vi "main5-2.vi"() -> ()   [LabVIEW 2018]
uses:
  <vilib>/Utility/file.llb/Write Delimited Spreadsheet (string).vi
panel:
  in  "备忘录保存路径":path
  out "光谱仪错误 2":errorcluster caption="光谱仪 R 错误"
  out "光谱仪错误":errorcluster caption="光谱仪 T 错误"
  in  "扫描模式":u16(ring)=2 items=["Norm/Hold", "Norm/Auto", "MID", "HIGH1", "HIGH2", "HIGH3", "Normal"]
  in  "终止波长":dbl=1542.0 caption="终止波长(nm)" format="%#_13g"
  in  "起始波长":dbl=1522.0 caption="起始波长(nm)" format="%#_13g"
  out "R中心波长-时间":waveform(dbl)(graph)
  out "T中心波长-时间":waveform(dbl)(graph)
  in  "T X dB":dbl=1.0 format="%#_13g"
  in  "保存路径R":path=path "C:/Users/Administrator/Desktop/超高温FBG实验程序/data/guangpuyi.txt" caption="R 光谱数据保存路径"
  in  "保存":bool
  in  "保存路径T":path=path "C:/Users/Administrator/Desktop/超高温FBG实验程序/data/guangpuyi.txt" caption="T 光谱数据保存路径"
  out "波峰带宽":dbl format="%.4f"
  out "Data X Value":dbl[](array[numeric]) format="%.4f"
  out "反射谱":T1(graph)
  out "R中心波长":dbl format="%.4f"
  out "波谷带宽":dbl format="%.4f"
  out "Data X Value":dbl[](array[numeric]) format="%.4f"
  out "采样点数":i32
  out "透射谱":T1(graph)
  out "T中心波长":dbl format="%.4f"
  in  "光谱仪 R":refnum<visa-resource-name>="光谱仪"
  in  "停止":bool
  in  "采集间隔":u32=30000 caption="采集间隔(ms)"
  in  "光谱仪 T":refnum<visa-resource-name>="光谱仪"
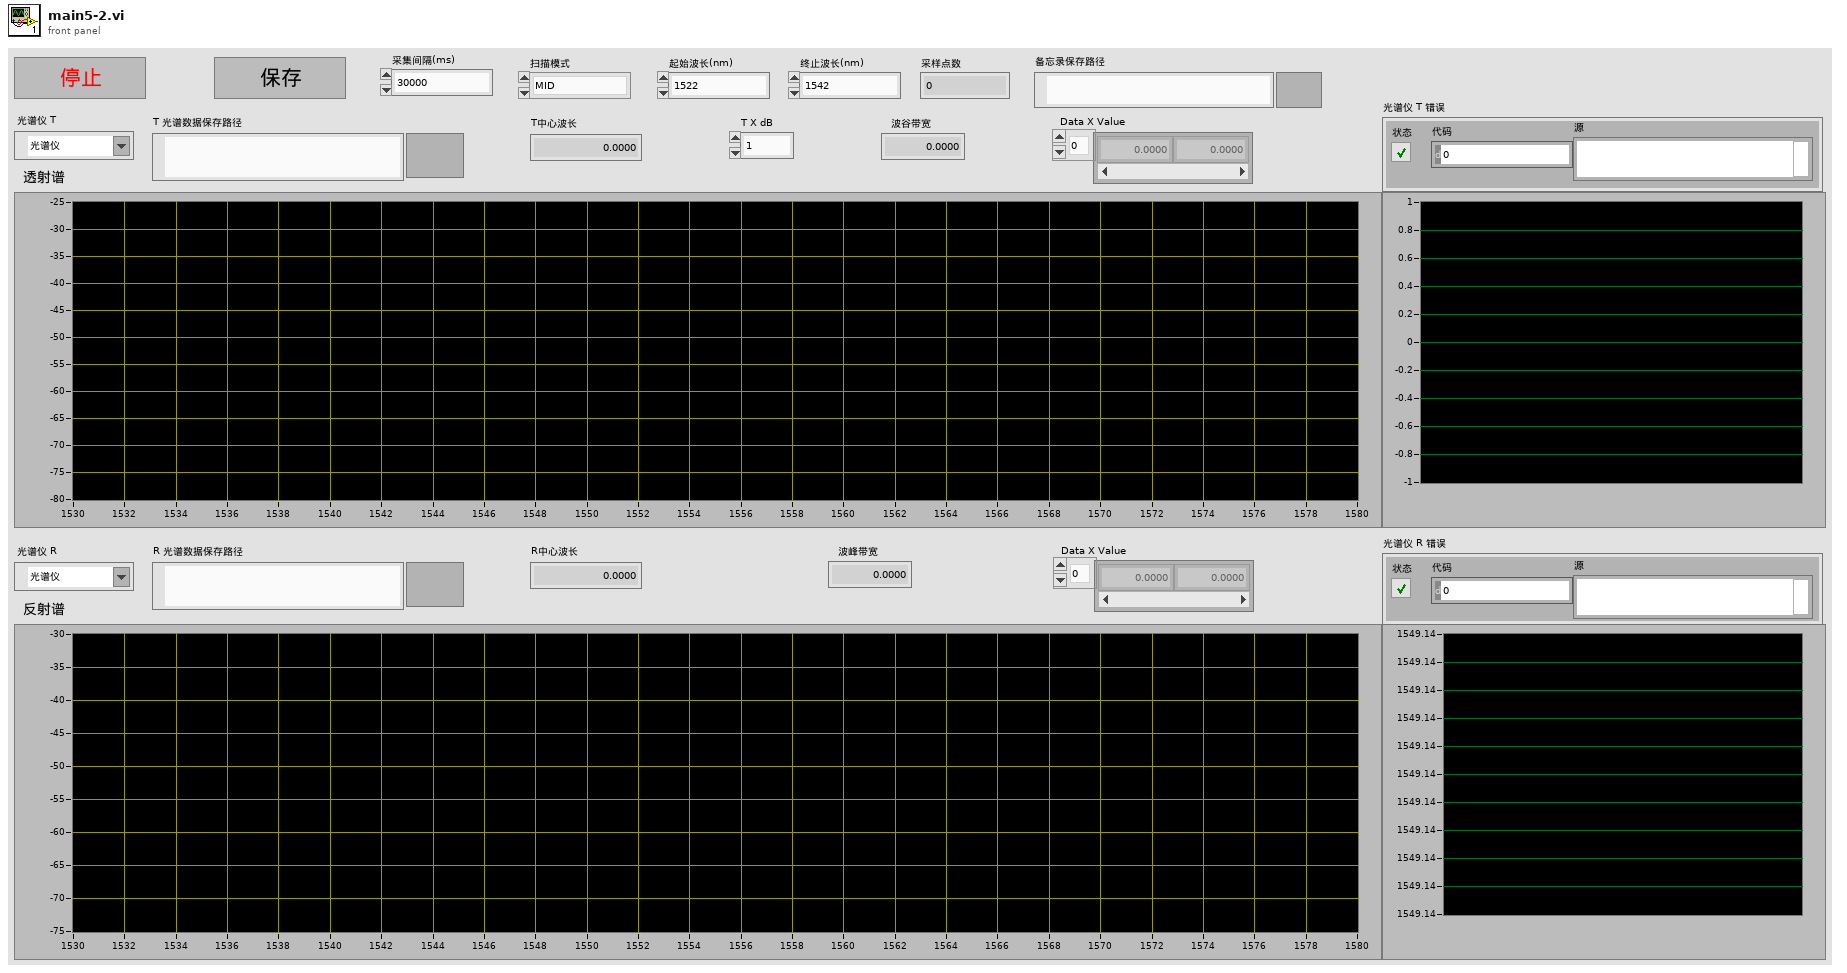
[diagram p1: front panel]
types:
  T1 = cluster{"Data X Value":dbl[], "Data Y Value":dbl[]}
  T2 = enum16{"open", "replace", "create", "open or create", "replace or create", "replace or create with confirmation"}
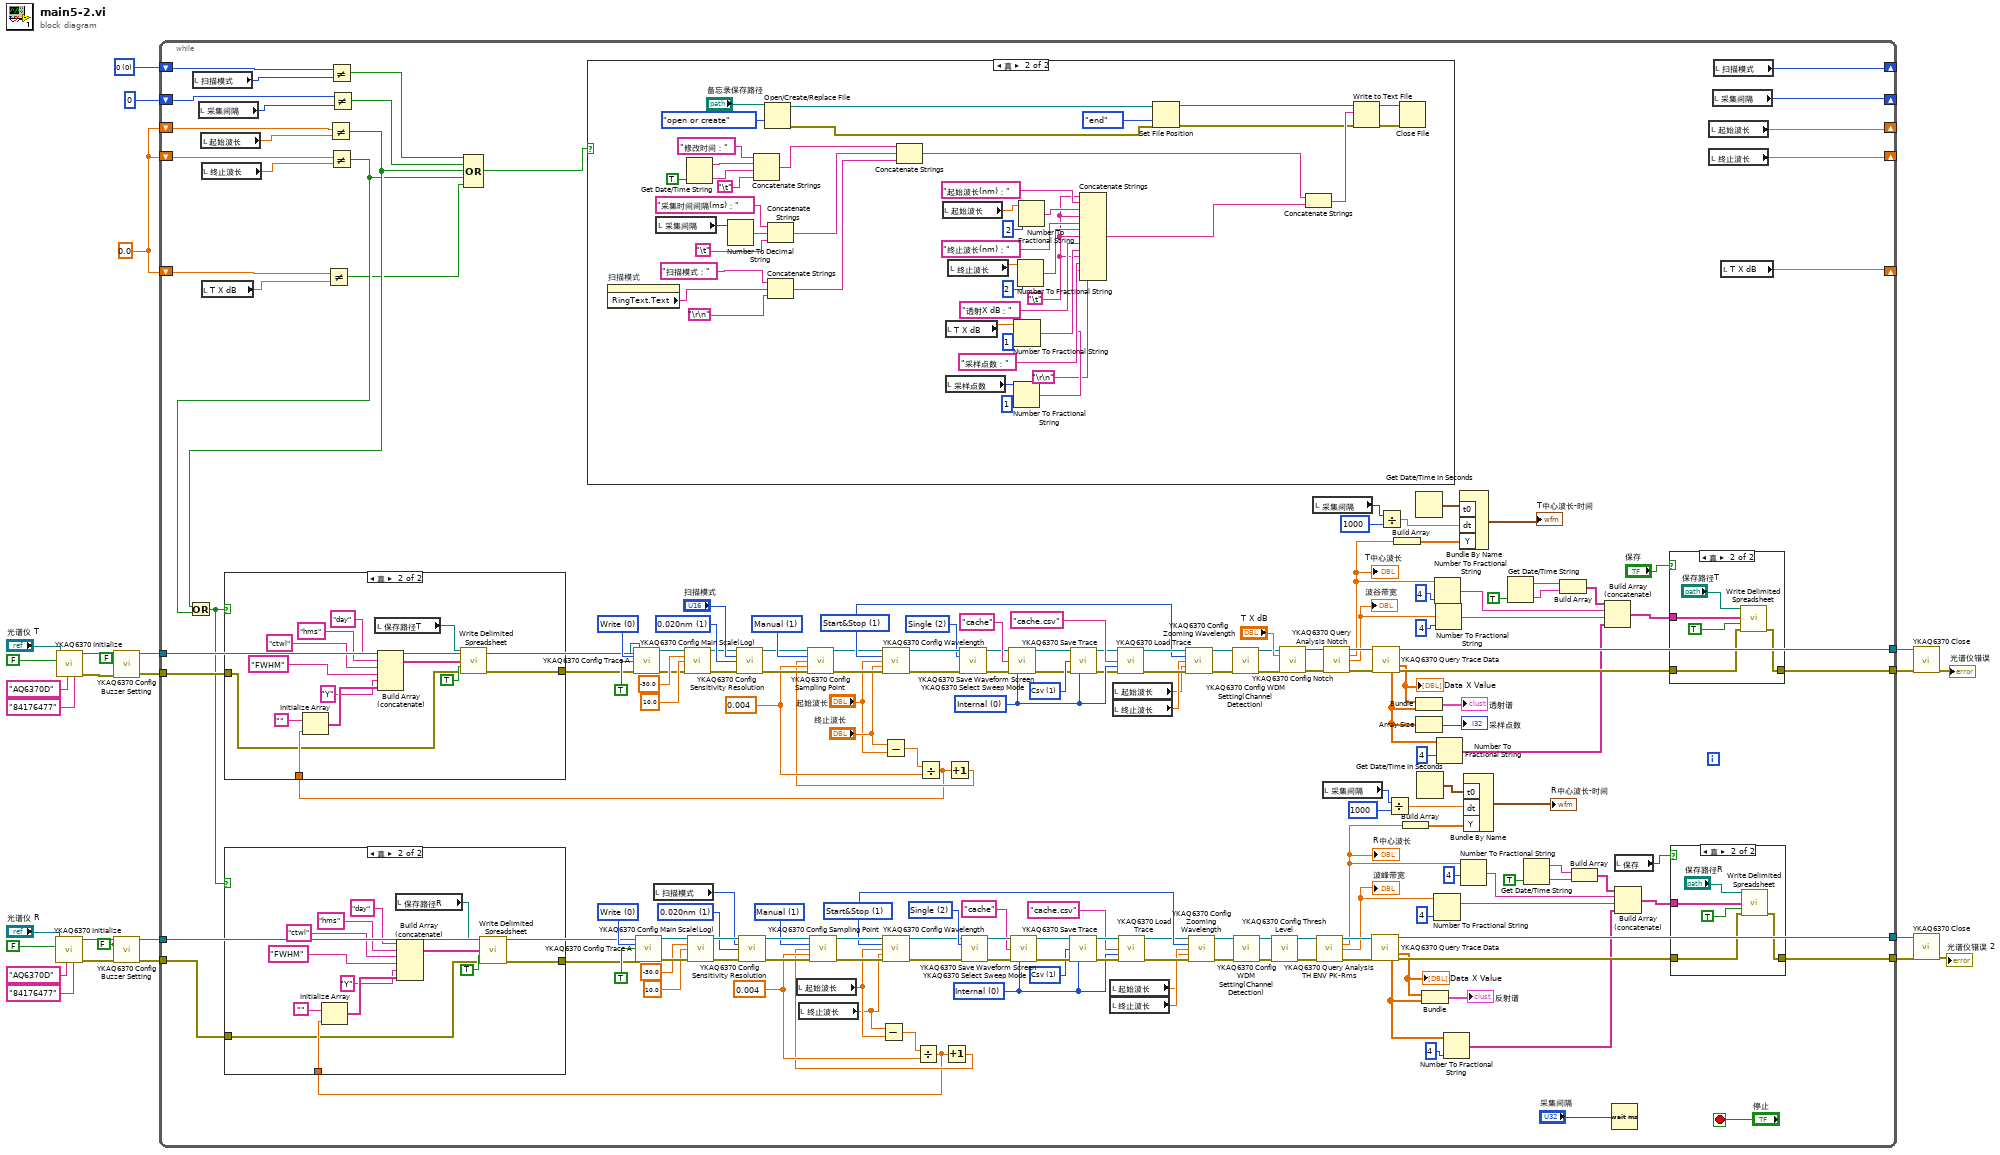
[diagram p0: block diagram]
diagram:
  w5 = u16 0 items=["0"]
  w6 = 0.0
  w12 = FALSE ("Click (T: ON)")
  w27 = FALSE ("Click (T: ON)")
  n1 = call "YKAQ6370 Initialize.vi"("Password (empty)"="84176477", "User Name (anonymous)"="AQ6370D", "ID Query? (T: Yes)"=FALSE, "VISA resource name"="光谱仪 R") -> ("error out"=w13:errorcluster, "VISA resource name out"=w14:refnum<visa-resource-name>)  [unwired: 6 in]
  n2 = call "YKAQ6370 Initialize.vi"("Password (empty)"="84176477", "User Name (anonymous)"="AQ6370D", "ID Query? (T: Yes)"=FALSE, "VISA resource name"="光谱仪 T") -> ("error out"=w26:errorcluster, "VISA resource name out"=w25:refnum<visa-resource-name>)  [unwired: 6 in]
  n3 = call "YKAQ6370 Config Buzzer Setting.vi"("VISA resource name"=w25, "Click (T: ON)"=w27, "Warning (T: ON)"=w27, "error in (no error)"=w26) -> ("VISA resource name out"=w20:refnum<visa-resource-name>, "error out"=w19:errorcluster)  [unwired: 10 in]
  n4 = call "YKAQ6370 Config Buzzer Setting.vi"("VISA resource name"=w14, "Click (T: ON)"=w12, "Warning (T: ON)"=w12, "error in (no error)"=w13) -> ("VISA resource name out"=w11:refnum<visa-resource-name>, "error out"=w10:errorcluster)  [unwired: 10 in]
  n5 = while {
    tunnel: w20 -> [w53]
    tunnel: w19 -> [w55]
    tunnel: w11 -> [w49]
    tunnel: w10 -> [w50]
    tunnel: [w33] -> w7
    shift-right: [w60] -> _
    shift-left: w6 -> [w67]
    shift-right: [w61] -> _
    shift-left: w6 -> [w69]
    shift-right: [w59] -> _
    shift-left: w6 -> [w71]
    shift-right: [w62] -> _
    shift-left: u32 0 -> [w72]
    shift-right: [w63] -> _
    shift-left: w5 -> [w75]
    tunnel: [w32] -> w3
    tunnel: [w31] -> w2
    tunnel: [w30] -> w1
    stop <- "停止" stop-if-true
    w144 = u16 1 items=["Bin", "Csv"] ("File Type (0: Bin)")
    w143 = u16 0 items=["Internal", "External"] ("Current Drive (0: Internal)")
    w154 = u16 1 items=["Center&Span", "Start&Stop"] ("Range Sw (0: Center&Span)")
    w157 = u16 1 items=["Auto", "Manual"] ("Sampling Point (0: Auto)")
    w161 = u16 1 items=["", "0.020nm", "0.050nm", "0.100nm", "0.200nm", "0.500nm", "1.000nm", "2.000nm", "4GHz", "10GHz", "20GHz", "40GHz", "100GHz", "200GHz", "400GHz"] ("Resolution (6: 1.000nm)")
    w94 = 0.004 ("Sample Interval (0.200)")
    w92 = u16 0 items=["Write", "Fix", "Max Hold", "Min Hold", "Roll Average"] ("Trace A ATTR  (0: Write)")
    w170 = u16 2 items=["Auto", "Repeat", "Single", "Stop", "Segment Measure"] ("Action Select (3: Stop)")
    w199 = u16 1 items=["Bin", "Csv"] ("File Type (0: Bin)")
    w200 = u16 0 items=["Internal", "External"] ("Current Drive (0: Internal)")
    w189 = u16 1 items=["Center&Span", "Start&Stop"] ("Range Sw (0: Center&Span)")
    w186 = u16 1 items=["Auto", "Manual"] ("Sampling Point (0: Auto)")
    w181 = u16 1 items=["", "0.020nm", "0.050nm", "0.100nm", "0.200nm", "0.500nm", "1.000nm", "2.000nm", "4GHz", "10GHz", "20GHz", "40GHz", "100GHz", "200GHz", "400GHz"] ("Resolution (6: 1.000nm)")
    w97 = 0.004 ("Sample Interval (0.200)")
    w184 = u16 0 items=["Write", "Fix", "Max Hold", "Min Hold", "Roll Average"] ("Trace A ATTR  (0: Write)")
    w171 = u16 2 items=["Auto", "Repeat", "Single", "Stop", "Segment Measure"] ("Action Select (3: Stop)")
    n6 = local read "扫描模式"() -> (w74:u16)
    n7 = local read "采集间隔"() -> (w73:u32)
    n8 = local read "起始波长"() -> (w70:dbl)
    n9 = local read "终止波长"() -> (w68:dbl)
    n10 = local read "T X dB"() -> (w66:dbl)
    n11 = Not Equal?(x=w67, y=w66) -> (x != y?=w34:bool)
    n12 = Not Equal?(x=w71, y=w70) -> (x != y?=w58:bool)
    n13 = Not Equal?(x=w75, y=w74) -> (x != y?=w65:bool)
    n14 = Not Equal?(x=w69, y=w68) -> (x != y?=w57:bool)
    n15 = Or(x=w58, y=w57) -> (x .or. y?=w47:bool)
    n16 = Not Equal?(x=w72, y=w73) -> (x != y?=w64:bool)
    n17 = Compound Arithmetic op=OR ("复合运算")(w65, w64, w58, w57, w34) -> (w48:bool)
    n18 = case shown="真" w48 {
      frame False {
      }
      frame True {
        w239 = "\t"
        n19 = property on="扫描模式" class="Ring (严格)"() -> ("RingText.Text"=w240:string)  [unwired: 2 in, 2 out]
        n20 = local read "采集间隔"() -> (w268:u32)
        n21 = Get Date/Time String(want seconds? (F)=TRUE ("需要秒？(F)")) -> (date string=w271:string, time string=w270:string)  [unwired: 2 in]
        n22 = Number To Decimal String(number=w268) -> (decimal integer string=w267:string)  [unwired: 1 in]
        n23 = Concatenate Strings("修改时间：" ("元素"), w271, w270, "\t") -> (w262:string)
        n24 = Open/Create/Replace File(file path (use dialog)="备忘录保存路径", operation (0:open)=T2."open or create" ("操作(0:open)")) -> (refnum out=w276:refnum<file>, error out=w242:errorcluster)  [unwired: 4 in, 1 out]
        n25 = Concatenate Strings("采集时间间隔(ms)：", w267, "\t") -> (w261:string)
        n26 = Concatenate Strings("扫描模式：", w240, "\r\n") -> (w260:string)
        n27 = Concatenate Strings(w262, w261, w260) -> (w247:string)
        n28 = local read "起始波长"() -> (w259:dbl)
        n29 = local read "T X dB"() -> (w255:dbl)
        n30 = local read "采样点数"() -> (w236:i32)
        n31 = local read "终止波长"() -> (w256:dbl)
        n32 = Number To Fractional String(number=w236, precision (6)=i16 1 ("精度(6)")) -> (F-format string=w235:string)  [unwired: 2 in]
        n33 = Number To Fractional String(number=w255, precision (6)=i16 1 ("精度(6)")) -> (F-format string=w248:string)  [unwired: 2 in]
        n34 = Number To Fractional String(number=w256, precision (6)=i16 2 ("精度(6)")) -> (F-format string=w250:string)  [unwired: 2 in]
        n35 = Number To Fractional String(number=w259, precision (6)=i16 2 ("精度(6)")) -> (F-format string=w252:string)  [unwired: 2 in]
        n36 = Concatenate Strings(w239, "起始波长(nm)：", w252, w239, "终止波长(nm)：", w250, w239, "透射X dB：", w248, w239, "采样点数：" ("字符串"), w235, "\r\n") -> (w246:string)
        n37 = Set File Position(refnum=w276, from (0:start)=enum16{"start", "end", "current"}."end" ("自（0:起始）"), error in=w242) -> (refnum out=w274:refnum<file>, error out=w241:errorcluster)  [unwired: 1 in]
        n38 = Concatenate Strings(w247, w246) -> (w245:string)
        n39 = Write to Text File(file (use dialog)=w274, text=w245, error in=w241) -> (refnum out=w244:refnum<file>, error out=w243:errorcluster)  [unwired: 1 in, 1 out]
        n40 = Close File(refnum=w244, error in=w243) -> ()  [unwired: 2 out]
      }
    }
    n41 = local read "扫描模式"() -> (w91:u16)
    n42 = local read "起始波长"() -> (w44:dbl)
    n43 = local read "终止波长"() -> (w43:dbl)
    n44 = Subtract(x=w43, y=w44) -> (x-y=w95:dbl)
    n45 = Subtract(x="终止波长", y="起始波长") -> (x-y=w98:dbl)
    n46 = Divide(x=w95, y=w94) -> (x/y=w52:dbl)
    n47 = case shown="真" w47 {
      tunnel: w52 -> [_ w210]
      tunnel: [w206 w209] -> w51
      tunnel: w50 -> [w206 w208]
      frame False {
      }
      frame True {
        n48 = Initialize Array("", w210) -> (w212:string[])
        n49 = local read "保存路径R"() -> (w211:path)
        n50 = Build Array (concatenate)("day" ("元素"), "hms" ("元素"), "ctwl" ("元素"), "FWHM" ("元素"), "Y" ("元素"), w212) -> (w219:string[])
        n51 = call-poly <vilib>:"Write Delimited Spreadsheet.vi"("file path (dialog if empty)"=w211, "1D data"=w219, "append to file? (new file:F)"=TRUE, "error in (no error)"=w208) -> ("error out"=w209:errorcluster)  [unwired: 10 in, 1 out]
      }
    }
    n52 = call "YKAQ6370 Config Trace A.vi"("VISA resource name"=w49, "Trace A ATTR  (0: Write)"=w92, "Disp / Blank (T: Disp)"=TRUE, "error in (no error)"=w51) -> ("VISA resource name out"=w165:refnum<visa-resource-name>, "error out"=w168:errorcluster)  [unwired: 10 in]
    n53 = call "YKAQ6370 Config Main Scale(Log).vi"("VISA resource name"=w165, "Reference Level (-10.0)"=-30.0, "Log Scale (10.0)"=10.0, "error in (no error)"=w168) -> ("VISA resource name out"=w164:refnum<visa-resource-name>, "error out"=w167:errorcluster)  [unwired: 10 in]
    n54 = call "YKAQ6370 Config Sensitivity Resolution.vi"("VISA resource name"=w164, "Sensitivity (1: Norm/Auto)"=w91, "Resolution (6: 1.000nm)"=w161, "error in (no error)"=w167) -> ("VISA resource name out"=w163:refnum<visa-resource-name>, "error out"=w166:errorcluster)  [unwired: 10 in]
    n55 = Divide(x=w98, y=w97) -> (x/y=w56:dbl)
    n56 = case shown="真" w47 {
      tunnel: w56 -> [_ w225]
      tunnel: w55 -> [w220 w223]
      tunnel: [w220 w222] -> w54
      frame False {
      }
      frame True {
        n57 = Initialize Array("", w225) -> (w224:string[])
        n58 = local read "保存路径T"() -> (w232:path)
        n59 = Build Array (concatenate)("day" ("元素"), "hms" ("元素"), "ctwl" ("元素"), "FWHM" ("元素"), "Y" ("元素"), w224) -> (w233:string[])
        n60 = call-poly <vilib>:"Write Delimited Spreadsheet.vi"("file path (dialog if empty)"=w232, "1D data"=w233, "append to file? (new file:F)"=TRUE, "error in (no error)"=w223) -> ("error out"=w222:errorcluster)  [unwired: 10 in, 1 out]
      }
    }
    n61 = call "YKAQ6370 Config Trace A.vi"("VISA resource name"=w53, "Trace A ATTR  (0: Write)"=w184, "Disp / Blank (T: Disp)"=TRUE, "error in (no error)"=w54) -> ("VISA resource name out"=w176:refnum<visa-resource-name>, "error out"=w173:errorcluster)  [unwired: 10 in]
    n62 = call "YKAQ6370 Config Main Scale(Log).vi"("VISA resource name"=w176, "Reference Level (-10.0)"=-30.0, "Log Scale (10.0)"=10.0, "error in (no error)"=w173) -> ("VISA resource name out"=w177:refnum<visa-resource-name>, "error out"=w174:errorcluster)  [unwired: 10 in]
    n63 = call "YKAQ6370 Config Sensitivity Resolution.vi"("VISA resource name"=w177, "Sensitivity (1: Norm/Auto)"="扫描模式", "Resolution (6: 1.000nm)"=w181, "error in (no error)"=w174) -> ("VISA resource name out"=w178:refnum<visa-resource-name>, "error out"=w175:errorcluster)  [unwired: 10 in]
    n64 = Increment(x=w52) -> (x+1=w93:dbl)
    n65 = call "YKAQ6370 Config Sampling Point.vi"("VISA resource name"=w163, "Sampling Point (0: Auto)"=w157, "Sampling Point (5501)"=w93, "Sample Interval (0.200)"=w94, "error in (no error)"=w166) -> ("VISA resource name out"=w162:refnum<visa-resource-name>, "error out"=w169:errorcluster)  [unwired: 9 in]
    n66 = call "YKAQ6370 Config Wavelength.vi"("VISA resource name"=w162, "Range Sw (0: Center&Span)"=w154, "Center/Start (1150.000)"=w44, "Span/Stop  (1100.000)"=w43, "error in (no error)"=w169) -> ("VISA resource name out"=w156:refnum<visa-resource-name>, "error out"=w155:errorcluster)  [unwired: 9 in]
    n67 = Increment(x=w56) -> (x+1=w96:dbl)
    n68 = call "YKAQ6370 Config Sampling Point.vi"("VISA resource name"=w178, "Sampling Point (0: Auto)"=w186, "Sampling Point (5501)"=w96, "Sample Interval (0.200)"=w97, "error in (no error)"=w175) -> ("VISA resource name out"=w179:refnum<visa-resource-name>, "error out"=w172:errorcluster)  [unwired: 9 in]
    n69 = call "YKAQ6370 Config Wavelength.vi"("VISA resource name"=w179, "Range Sw (0: Center&Span)"=w189, "Center/Start (1150.000)"="起始波长", "Span/Stop  (1100.000)"="终止波长", "error in (no error)"=w172) -> ("VISA resource name out"=w187:refnum<visa-resource-name>, "error out"=w188:errorcluster)  [unwired: 9 in]
    n70 = call "YKAQ6370 Select Sweep Mode.vi"("VISA resource name"=w187, "Action Select (3: Stop)"=w171, "error in (no error)"=w188) -> ("VISA resource name out"=w192:refnum<visa-resource-name>, "error out"=w193:errorcluster)  [unwired: 11 in]
    n71 = call "YKAQ6370 Select Sweep Mode.vi"("VISA resource name"=w156, "Action Select (3: Stop)"=w170, "error in (no error)"=w155) -> ("VISA resource name out"=w151:refnum<visa-resource-name>, "error out"=w150:errorcluster)  [unwired: 11 in]
    n72 = call "YKAQ6370 Save Waveform Screen.vi"("VISA resource name"=w192, "File Name (empty)"="cache", "error in (no error)"=w193, "Current Drive (0: Internal)"=w200) -> ("VISA resource name out"=w194:refnum<visa-resource-name>, "error out"=w190:errorcluster)  [unwired: 10 in]
    n73 = call "YKAQ6370 Save Waveform Screen.vi"("VISA resource name"=w151, "File Name (empty)"="cache", "error in (no error)"=w150, "Current Drive (0: Internal)"=w143) -> ("VISA resource name out"=w149:refnum<visa-resource-name>, "error out"=w153:errorcluster)  [unwired: 10 in]
    n74 = call "YKAQ6370 Save Trace.vi"("VISA resource name"=w149, "File Type (0: Bin)"=w144, "error in (no error)"=w153, "Current Drive (0: Internal)"=w143) -> ("VISA resource name out"=w148:refnum<visa-resource-name>, "error out"=w152:errorcluster)  [unwired: 10 in]
    n75 = call "YKAQ6370 Save Trace.vi"("VISA resource name"=w194, "File Type (0: Bin)"=w199, "error in (no error)"=w190, "Current Drive (0: Internal)"=w200) -> ("VISA resource name out"=w195:refnum<visa-resource-name>, "error out"=w191:errorcluster)  [unwired: 10 in]
    n76 = local read "起始波长"() -> (w45:dbl)
    n77 = local read "终止波长"() -> (w46:dbl)
    n78 = local read "起始波长"() -> (w101:dbl)
    n79 = local read "终止波长"() -> (w102:dbl)
    n80 = call "YKAQ6370 Load Trace.vi"("VISA resource name"=w195, "File Name (empty)"="cache.csv", "Current Drive (0: Internal)"=w200, "error in (no error)"=w191) -> ("VISA resource name out"=w196:refnum<visa-resource-name>, "error out"=w197:errorcluster)  [unwired: 10 in]
    n81 = call "YKAQ6370 Load Trace.vi"("VISA resource name"=w148, "File Name (empty)"="cache.csv", "Current Drive (0: Internal)"=w143, "error in (no error)"=w152) -> ("VISA resource name out"=w147:refnum<visa-resource-name>, "error out"=w146:errorcluster)  [unwired: 10 in]
    n82 = call "YKAQ6370 Config Zooming Wavelength.vi"("VISA resource name"=w196, "Range Sw (0: Center&Span)"=w189, "Span/Stop (1100.000)"=w102, "Center/Start(1150.000)"=w101, "error in (no error)"=w197) -> ("VISA resource name out"=w202:refnum<visa-resource-name>, "error out"=w203:errorcluster)  [unwired: 9 in]
    n83 = call "YKAQ6370 Config Zooming Wavelength.vi"("VISA resource name"=w147, "Range Sw (0: Center&Span)"=w154, "Span/Stop (1100.000)"=w46, "Center/Start(1150.000)"=w45, "error in (no error)"=w146) -> ("VISA resource name out"=w141:refnum<visa-resource-name>, "error out"=w140:errorcluster)  [unwired: 9 in]
    n84 = call "YKAQ6370 Config WDM Setting(Channel Detection).vi"("VISA resource name"=w202, "error in (no error)"=w203) -> ("VISA resource name out"=w127:refnum<visa-resource-name>, "error out"=w126:errorcluster)  [unwired: 12 in]
    n85 = call "YKAQ6370 Config WDM Setting(Channel Detection).vi"("VISA resource name"=w141, "error in (no error)"=w140) -> ("VISA resource name out"=w35:refnum<visa-resource-name>, "error out"=w41:errorcluster)  [unwired: 12 in]
    n86 = call "YKAQ6370 Config Thresh Level.vi"("VISA resource name"=w35, "error in (no error)"=w41) -> ("VISA resource name out"=w39:refnum<visa-resource-name>, "error out"=w42:errorcluster)  [unwired: 12 in]
    n87 = call "YKAQ6370 Config Notch.vi"("VISA resource name"=w127, "Thresh Level (3.00)"="T X dB", "error in (no error)"=w126) -> ("VISA resource name out"=w133:refnum<visa-resource-name>, "error out"=w132:errorcluster)  [unwired: 11 in]
    n88 = local read "采集间隔"() -> (w85:u32)
    n89 = call "YKAQ6370 Query Analysis TH ENV PK-Rms.vi"("VISA resource name"=w39, "error in (no error)"=w42) -> ("VISA resource name out"=w38:refnum<visa-resource-name>, "Center WL"=w37:dbl, "Spec Width"=w36:dbl, "error out"=w40:errorcluster)  [unwired: 9 in, 1 out]
    "R中心波长" <- w37
    "波峰带宽" <- w36
    n90 = local read "采集间隔"() -> (w81:u32)
    n91 = call "YKAQ6370 Query Analysis Notch.vi"("VISA resource name"=w133, "error in (no error)"=w132) -> ("VISA resource name out"=w135:refnum<visa-resource-name>, "Center WL"=w89:dbl, "Notch Width"=w113:dbl, "error out"=w134:errorcluster)  [unwired: 10 in]
    "T中心波长" <- w89
    "波谷带宽" <- w113
    n92 = call "YKAQ6370 Query Trace Data.vi"("VISA resource name"=w38, "error in (no error)"=w40) -> ("VISA resource name out"=w33:refnum<visa-resource-name>, "Data X Value"=w76:dbl[], "Data Y Value"=w128:dbl[], "error out"=w116:errorcluster)  [unwired: 7 in, 3 out]
    "Data X Value" <- w76
    n93 = call "YKAQ6370 Query Trace Data.vi"("VISA resource name"=w135, "error in (no error)"=w134) -> ("VISA resource name out"=w30:refnum<visa-resource-name>, "Data X Value"=w77:dbl[], "Data Y Value"=w136:dbl[], "error out"=w117:errorcluster)  [unwired: 7 in, 3 out]
    "Data X Value" <- w77
    n94 = Divide(x=w85, y=u32 1000) -> (x/y=w83:dbl)
    n95 = Divide(x=w81, y=u32 1000) -> (x/y=w79:dbl)
    n96 = Build Array(w89) -> (w90:dbl[])
    n97 = Build Array(w37) -> (w86:dbl[])
    n98 = Get Date/Time In Seconds() -> (seconds since 1Jan1904=w87:timestamp)
    n99 = Bundle("Data X Value"=w77, "Data Y Value"=w136) -> (→"透射谱":T1)  [unwired: 1 in]
    n100 = Array Size(array=w136) -> (size(s)=→"采样点数":i32)
    n101 = Get Date/Time In Seconds() -> (seconds since 1Jan1904=w82:timestamp)
    n102 = Bundle("Data X Value"=w76, "Data Y Value"=w128) -> (→"反射谱":T1)  [unwired: 1 in]
    n103 = Number To Fractional String(number=w36, precision (6)=i16 4 ("精度(6)")) -> (F-format string=w118:string)  [unwired: 2 in]
    n104 = Number To Fractional String(number=w89, precision (6)=i16 4 ("精度(6)")) -> (F-format string=w122:string)  [unwired: 2 in]
    n105 = Number To Fractional String(number=w113, precision (6)=i16 4 ("精度(6)")) -> (F-format string=w121:string)  [unwired: 2 in]
    n106 = Number To Fractional String(number=w136, precision (6)=i16 4 ("精度(6)")) -> (F-format string=w29:string[])  [unwired: 2 in]
    n107 = Number To Fractional String(number=w128, precision (6)=i16 4 ("精度(6)")) -> (F-format string=w28:string[])  [unwired: 2 in]
    n108 = Bundle By Name("t0"=w87, "dt"=w83, "Y"=w90) -> (→"T中心波长-时间":waveform(dbl))  [unwired: 1 in]
    n109 = Number To Fractional String(number=w37, precision (6)=i16 4 ("精度(6)")) -> (F-format string=w119:string)  [unwired: 2 in]
    n110 = Bundle By Name("t0"=w82, "dt"=w79, "Y"=w86) -> (→"R中心波长-时间":waveform(dbl))  [unwired: 1 in]
    n111 = Get Date/Time String(want seconds? (F)=TRUE ("需要秒？(F)")) -> (date string=w124:string, time string=w114:string)  [unwired: 2 in]
    n112 = Get Date/Time String(want seconds? (F)=TRUE ("需要秒？(F)")) -> (date string=w110:string, time string=w109:string)  [unwired: 2 in]
    n113 = Build Array(w124, w114) -> (w104:string[])
    n114 = Build Array(w110, w109) -> (w106:string[])
    n115 = Build Array (concatenate)(w104, w122, w121, w29) -> (w120:string[])
    n116 = Wait (ms)(milliseconds to wait="采集间隔") -> ()  [unwired: 1 out]
    n117 = local read "保存"() -> (w103:bool)
    n118 = Build Array (concatenate)(w106, w119, w118, w28) -> (w105:string[])
    n119 = case shown="真" "保存" {
      tunnel: w117 -> [w285 w286]
      tunnel: [w285 w290] -> w31
      tunnel: w120 -> [_ w287]
      frame False {
      }
      frame True {
        n120 = call-poly <vilib>:"Write Delimited Spreadsheet.vi"("file path (dialog if empty)"="保存路径T", "1D data"=w287, "append to file? (new file:F)"=TRUE, "error in (no error)"=w286) -> ("error out"=w290:errorcluster)  [unwired: 10 in, 1 out]
      }
    }
    n121 = case shown="真" w103 {
      tunnel: [w279 w284] -> w32
      tunnel: w116 -> [w279 w281]
      tunnel: w105 -> [_ w280]
      frame False {
      }
      frame True {
        n122 = call-poly <vilib>:"Write Delimited Spreadsheet.vi"("file path (dialog if empty)"="保存路径R", "1D data"=w280, "append to file? (new file:F)"=TRUE, "error in (no error)"=w281) -> ("error out"=w284:errorcluster)  [unwired: 10 in, 1 out]
      }
    }
    n123 = local read "起始波长"() -> (w59:dbl)
    n124 = local read "终止波长"() -> (w61:dbl)
    n125 = local read "采集间隔"() -> (w62:u32)
    n126 = local read "扫描模式"() -> (w63:u16)
    n127 = local read "T X dB"() -> (w60:dbl)
  }
  n128 = call "YKAQ6370 Close.vi"("error in (no error)"=w2, "VISA resource name"=w1) -> ("error out"=→"光谱仪错误":errorcluster)  [unwired: 9 in]
  n129 = call "YKAQ6370 Close.vi"("error in (no error)"=w3, "VISA resource name"=w7) -> ("error out"=→"光谱仪错误 2":errorcluster)  [unwired: 9 in]
